vi "Insert After.vi"(8 "error in (no error)":errorcluster, 11 "Test Configs In":T1) -> (0 "error out":errorcluster, 3 "Test Configs Out":T1)   [LabVIEW 2015]
doc: "Insert either a copied array element or default array element after the active element."
uses:
  Type Defs/Sequence Parameters Ref.ctl
  Type Defs/Sequence Parameters.ctl
  Type Defs/Target Type.ctl
  Type Defs/Variable Data Type.ctl
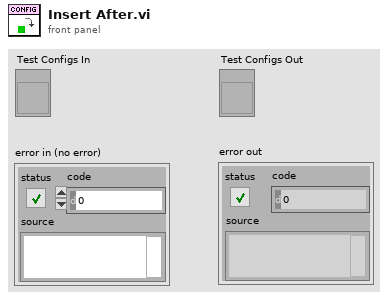
[diagram p1: front panel]
types:
  T1 = typedef "Sequence Parameters Ref.ctl" = refnum<vi>
  T2 = typedef "Sequence Parameters.ctl" = cluster{"Test Name":string, "Target":T3, "Host IP Address":string, "Target IP Address":string, "Shared Variable Host":enum16{"Target", "Host"}, "Shared Variable Writer":enum16{"Target", "Host"}, "Variable Data Type":T4, "# of Variables per Library":u16, "Update Rate (Hz)":dbl, "Read Rate (Hz)":dbl, "Floor":u32, "Ceiling":u32, "Delta":u32}
  T3 = typedef "Target Type.ctl" = enum16{"cRIO-9012", "cRIO-9014", "cRIO-9022", "cRIO-9023", "cRIO-9024", "cRIO-9025", "cRIO-9068", "cRIO-9073", "cRIO-9074", "cRIO-9075", "cRIO-9076", "cRIO-9081", "cRIO-9082", "myRIO-1900", "myRIO-1950", "PXI-8101", "PXI-8115", "PXI-8119", "PXI-8820", "PXIe-8100", "PXIe-8101", "PXIe-8133", "PXIe-8135", "PXIe-8820", "sbRIO-9605", "sbRIO-9606", "sbRIO-9623", "sbRIO-9626", "sbRIO-9633", "sbRIO-9636", "Unlisted (Linux-RT)", "Unlisted (PharLap)", "Unlisted (VxWorks)", "Windows Target"}
  T4 = typedef "Variable Data Type.ctl" = enum16{"U8", "U16", "U32", "U64", "I8", "I16", "I32", "I64", "Single", "Double", "Boolean", "String"}
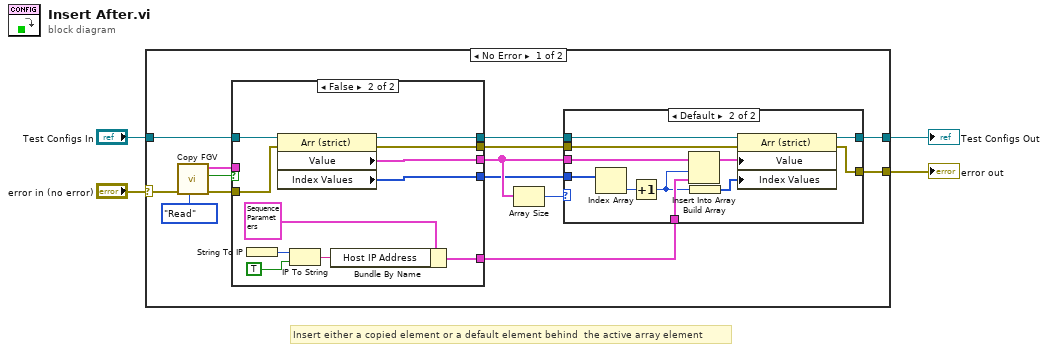
[diagram p0: block diagram]
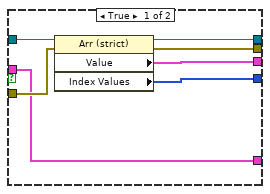
[diagram p3: hidden frame]
diagram:
  # "Insert either a copied element or a default element behind  the active array element"
  n1 = case shown="No Error" "error in (no error)" {
    selector: "error in (no error)" -> [w18 w50]
    tunnel: "Test Configs In" -> [w13 w51]
    tunnel: [w6 w51] -> w1
    tunnel: [w5 w50] -> w2
    frame No Error {
      n2 = call "Copy FGV.vi"("Mode"=enum16{"Enable Copy", "Disable Copy", "Read"}."Read", "error in (no error)"=w18) -> ("error out"=w14:errorcluster, "Copy Enabled? Out"=w16:bool, "Element to Read"=w15:T2)  [unwired: 7 in]
      n3 = case shown="False" w16 {
        tunnel: w15 -> [w32 _]
        tunnel: w14 -> [w37 w48]
        tunnel: w13 -> [w38 w49]
        tunnel: [w36 w42] -> w11
        tunnel: [w32 w43] -> w7
        tunnel: [w35 w41] -> w10
        tunnel: [w34 w40] -> w9
        tunnel: [w33 w39] -> w8
        frame True {
          n4 = property class="Arr (strict)"(reference=w38, error in=w37) -> (reference out=w36:T1, error out=w35:errorcluster, "Value"=w34:T2[], "Index Values"=w33:u32[])
        }
        frame False {
          n5 = String To IP() -> (0:w46:u32)  [unwired: 1 in]
          n6 = property class="Arr (strict)"(reference=w49, error in=w48) -> (reference out=w42:T1, error out=w41:errorcluster, "Value"=w40:T2[], "Index Values"=w39:u32[])
          n7 = IP To String(1:TRUE, 2:w46) -> (0:w44:string)
          n8 = Bundle By Name(cluster=T2 {"Test Name"="Unique Test Name", "Target"=enum."cRIO-9012", "Host IP Address"="0.0.0.0", "Target IP Address"="0.0.0.0", "Shared Variable Host"=enum."Target", "Shared Variable Writer"=enum."Target", "Variable Data Type"=enum."Double", "# of Variables per Library"=500, "Update Rate (Hz)"=1.0, "Read Rate (Hz)"=1.0, "Floor"=500, "Ceiling"=5000, "Delta"=500} ("Test Parameters"), "Host IP Address"=w44) -> (w43:T2)
        }
      }
      n9 = Array Size(array=w9) -> (size(s)=w12:i32)
      n10 = case shown="Default" w12 {
        tunnel: w8 -> [_ w31]
        tunnel: w11 -> [w20 w30]
        tunnel: w10 -> [w19 w29]
        tunnel: [w20 w27] -> w6
        tunnel: [w19 w26] -> w5
        tunnel: w7 -> [_ w24]
        tunnel: w9 -> [_ w21]
        frame 0 {
        }
        frame Default {
          n11 = Index Array(array=w31) -> (element=w25:u32)  [unwired: 1 in]
          n12 = Increment(x=w25) -> (x+1=w23:u32)
          n13 = Insert Into Array(array=w21, index=w23, new element=w24) -> (w28:T2[])
          n14 = Build Array(w23) -> (w22:u32[])
          n15 = property class="Arr (strict)"(reference=w30, error in=w29, "Value"=w28, "Index Values"=w22) -> (reference out=w27:T1, error out=w26:errorcluster)
        }
      }
    }
    frame Error {
    }
  }
  "Test Configs Out" <- w1
  "error out" <- w2
